vi "Hide AppBar.vi"(8 "error in (no error)":errorcluster, 10 "Stop AppBar? (T)":bool=TRUE, 11 "MainController in":refnum<class "MainController.lvclass">) -> (0 "error out":errorcluster, 3 "MainController out":refnum<class "MainController.lvclass">)   [LabVIEW 2012, in "Win8uiFramework.lvlib" / "MainController.lvclass"]
uses:
  MainController.lvclass
  MainController.lvclass/MainController.ctl
  Visibility Direction.ctl
  Visiblity States.ctl
  <vilib>/ActorFramework/Message Enqueuer/Message Enqueuer.lvclass/Message Enqueuer.ctl
  <vilib>/ActorFramework/Message Enqueuer/Message Enqueuer.lvclass
  Write AppBar Enqueuer.vi
  Write AppBar State.vi
  Read AppBar Enqueuer.vi
  Read AppBar State.vi
  <vilib>/ActorFramework/Message Enqueuer/Enqueue.vi
  <vilib>/ActorFramework/Message Priority Queue/Priority Enqueue.vi
  Remove From SubPanel Msg.lvclass
  <vilib>/ActorFramework/Stop Msg/Stop Msg.lvclass
  Win8uiFramework.lvlib
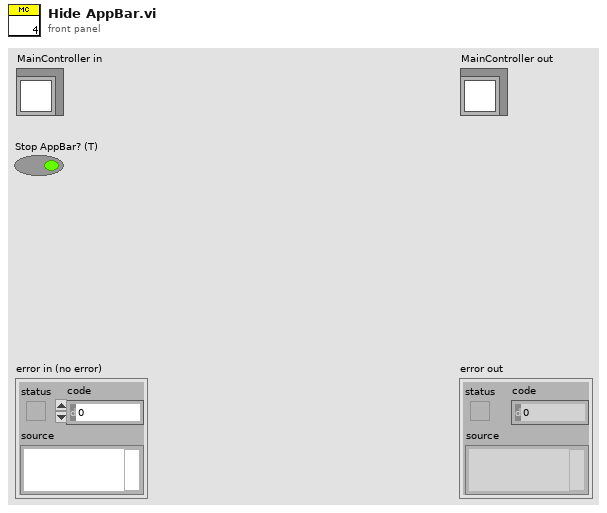
[diagram p1: front panel]
types:
  T1 = typedef "Win8uiFramework.lvlib/Visibility Direction.ctl" = enum16{"Show", "Hide"}
  T2 = typedef "Win8uiFramework.lvlib/MainController.lvclass/Visiblity States.ctl" = enum16{"Disabled", "Hidden - Unpopulated", "Hidden - Populated", "Visible"}
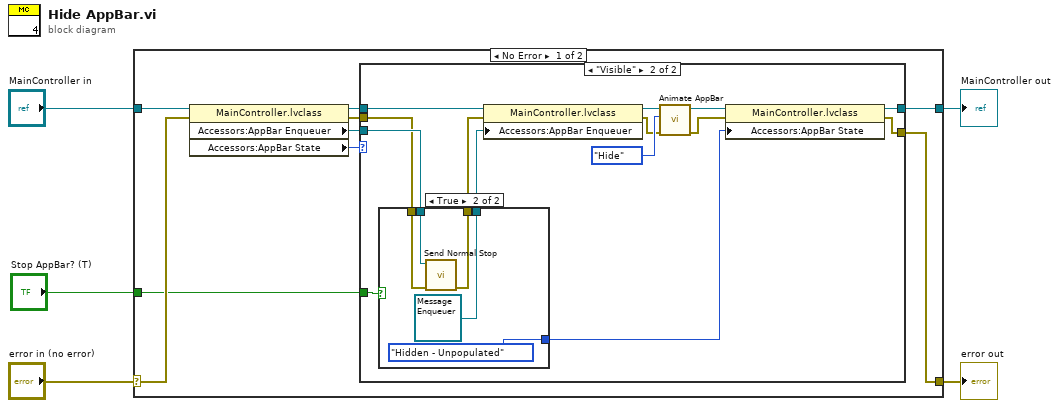
[diagram p0: block diagram]
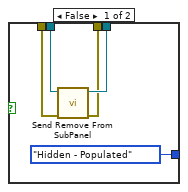
[diagram p3: hidden frame]
diagram:
  n1 = case shown="No Error" "error in (no error)" {
    selector: "error in (no error)" -> [w10 w42]
    tunnel: [w12 w42] -> w4
    tunnel: [w13 w41] -> w2
    tunnel: "MainController in" -> [w14 w41]
    tunnel: "Stop AppBar? (T)" -> [w7 _]
    frame No Error {
      n2 = property class="MainController.lvclass"(reference=w14, error in=w10) -> (reference out=w11:refnum<class "MainController.lvclass">, error out=w8:errorcluster, "Accessors:AppBar Enqueuer"=w9:refnum<class "Message Enqueuer.lvclass">, "Accessors:AppBar State"=w6:T2)
      n3 = case shown="\"Visible\"" w6 {
        tunnel: [w16 w20] -> w13
        tunnel: [w15 w18] -> w12
        tunnel: w11 -> [w16 w29]
        tunnel: w9 -> [_ w26]
        tunnel: w8 -> [w15 w25]
        tunnel: w7 -> [_ w22]
        frame Default {
        }
        frame "Visible" {
          n4 = case shown="True" w22 {
            tunnel: w26 -> [w35 w40]
            tunnel: w25 -> [w34 w39]
            tunnel: [w32 w38] -> w24
            tunnel: [w33 refnum<class "Message Enqueuer.lvclass"> refnum ("AppBar Enqueuer")] -> w23
            tunnel: [Visiblity_States."Hidden - Populated" ("Charm State") Visiblity_States."Hidden - Unpopulated" ("Charm State")] -> w17
            frame False {
              n5 = call "Send Remove From SubPanel.vi"("error in (no error)"=w34, "Message Enqueuer"=w35) -> ("error out"=w32:errorcluster, "Message Enqueuer out"=w33:refnum<class "Message Enqueuer.lvclass">)  [unwired: 8 in]
            }
            frame True {
              n6 = call <vilib>:"Send Normal Stop.vi"("error in (no error)"=w39, "Message Enqueuer"=w40) -> ("error out"=w38:errorcluster)  [unwired: 9 in]
            }
          }
          n7 = property class="MainController.lvclass"(reference=w29, error in=w24, "Accessors:AppBar Enqueuer"=w23) -> (reference out=w28:refnum<class "MainController.lvclass">, error out=w27:errorcluster)
          n8 = call-dynamic "Animate AppBar.vi"("error in (no error)"=w27, "Direction"=Visibility_Direction."Hide", "MainController in"=w28) -> ("error out"=w19:errorcluster, "MainController out"=w21:refnum<class "MainController.lvclass">)  [unwired: 7 in]
          n9 = property class="MainController.lvclass"(reference=w21, error in=w19, "Accessors:AppBar State"=w17) -> (reference out=w20:refnum<class "MainController.lvclass">, error out=w18:errorcluster)
        }
      }
    }
    frame Error {
    }
  }
  "error out" <- w4
  "MainController out" <- w2
